vi "SerialFrameProtocol_example.vi"() -> ()   [LabVIEW 2015]
uses:
  <vilib>/Instr/_visa.llb/VISA Flush IO Buffer Mask.ctl
  <vilib>/Instr/_visa.llb/VISA Set IO Buffer Mask.ctl
  <vilib>/Instr/_visa.llb/VISA Configure Serial Port (Instr).vi
panel:
  out "length 2":i32
  out "length":i32
  in  "VISA resource name":refnum<visa-resource-name>="COM8"
  out "buffer, NORMAL == read buffer unstuffing, NORMAL":bool
  out "size(s)":i32
  out "size(s)":i32
  out "Receiv Array":u8[](array[numeric])
  out "Send Array":u8[](array[numeric])
  out "Data2 (U16)":u16[](array[numeric])
  out "size(Data2)":i32
  out "size(Data1)":i32
  out "Data1 (I32)":i32[](array[numeric])
  out "B0":cluster{"iVal":i32, "fVal":sgl}
  out "buffer, HEX":string
  out "buffer, NORMAL":string
  out "buffer stuffing, HEX":string
  in  "Clear log":bool
  in  "CA":bool
  out "log":string
  in  "CL":bool
  in  "CZ":bool
  out "VISA Read counter":i32
  out "error IO":errorcluster
  out "VISA Read no error counter":i32
  in  "CN":bool
  in  "CY":bool
  in  "CB":bool
  out "CX Send array == AX read array":bool
  out "read buffer unstuffing, HEX":string
  out "read buffer unstuffing, NORMAL":string
  out "buffer stuffing, NORMAL":string
  out "read buffer RAW, HEX":string
  in  "stop":bool
  out "Counter":i32
  out "read buffer RAW, NORMAL":string="\n"
  in  "CX Send rand array":bool
  # "Serial Frame Protocol Test"
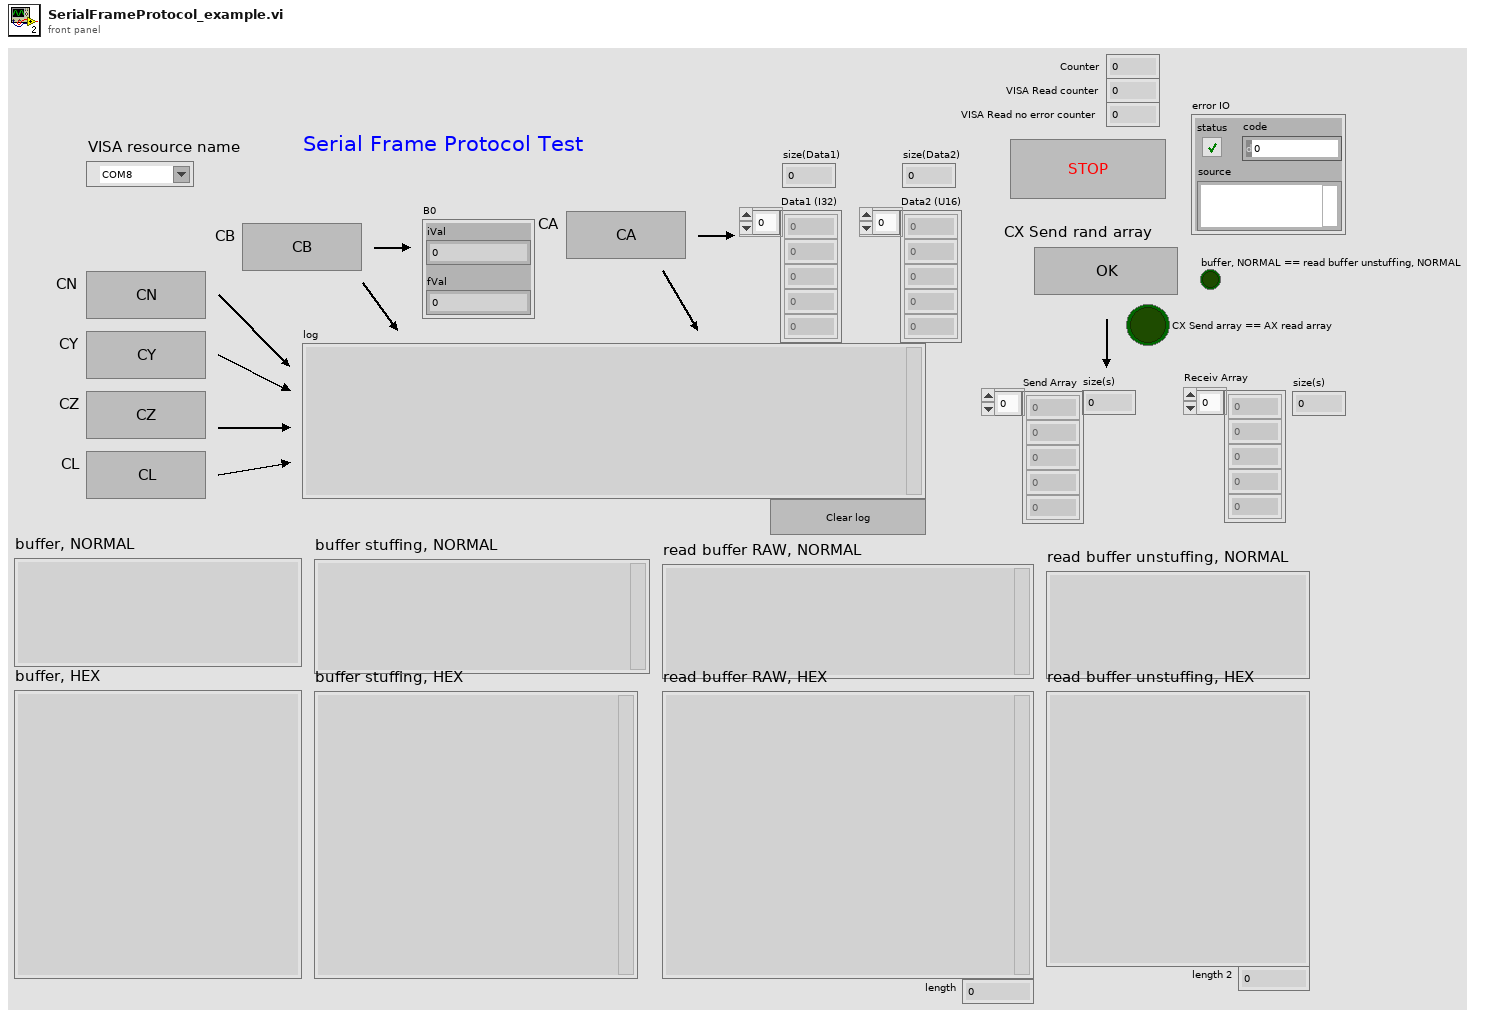
[diagram p1: front panel]
types:
  T1 = typedef "VISA Set IO Buffer Mask.ctl" = u16
  T2 = typedef "VISA Flush IO Buffer Mask.ctl" = u16
  T3 = enum16{"big-endian, network order", "native, host order", "little-endian"}
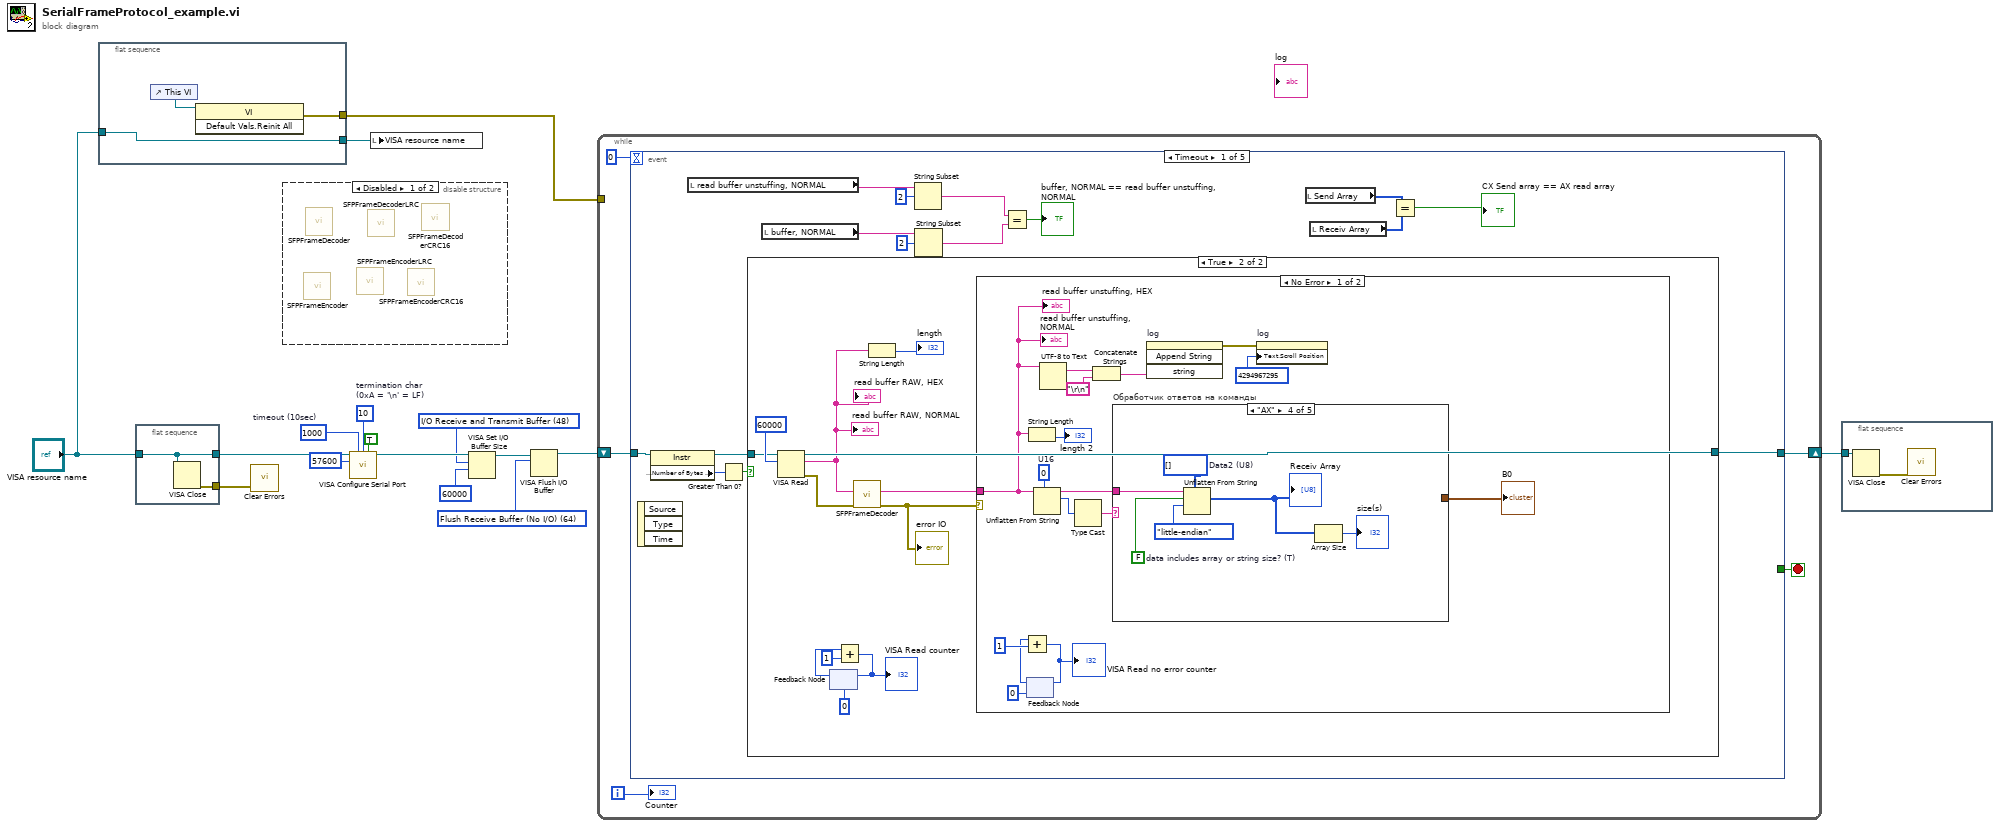
[diagram p0: block diagram]
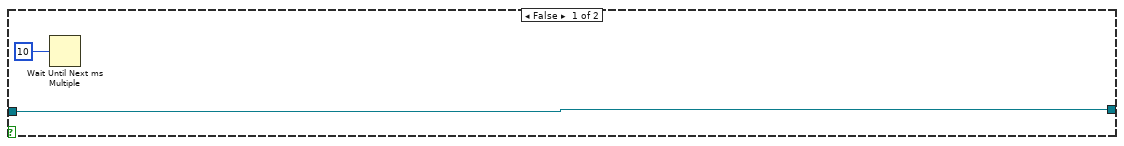
[diagram p2: hidden frame]
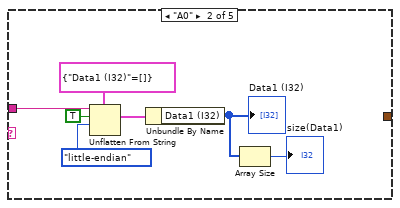
[diagram p4: hidden frame]
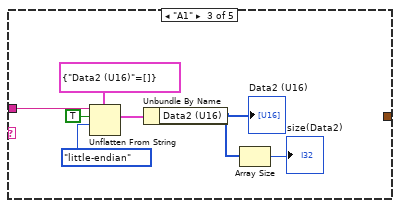
[diagram p5: hidden frame]
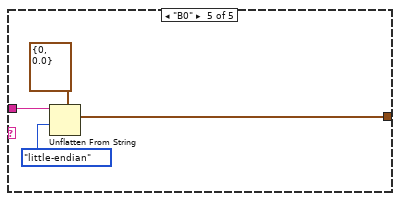
[diagram p6: hidden frame]
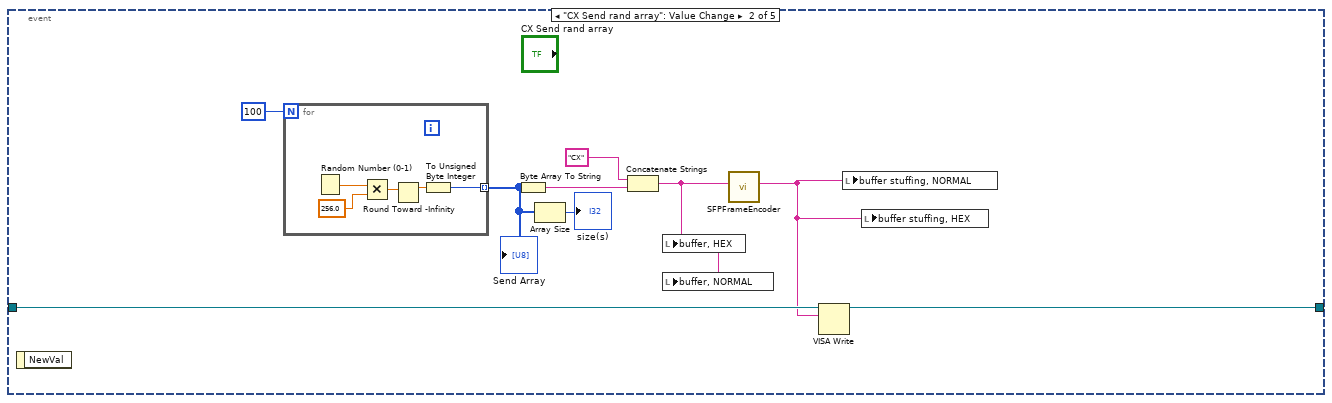
[diagram p8: hidden frame]
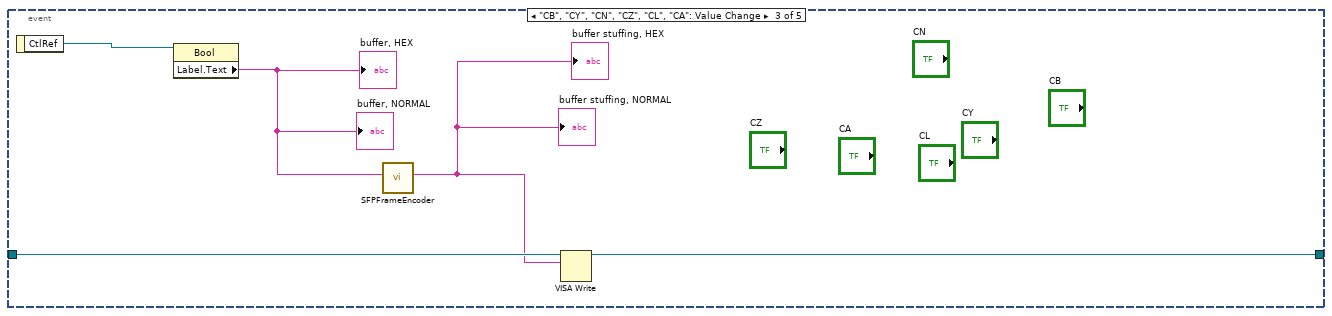
[diagram p9: hidden frame]
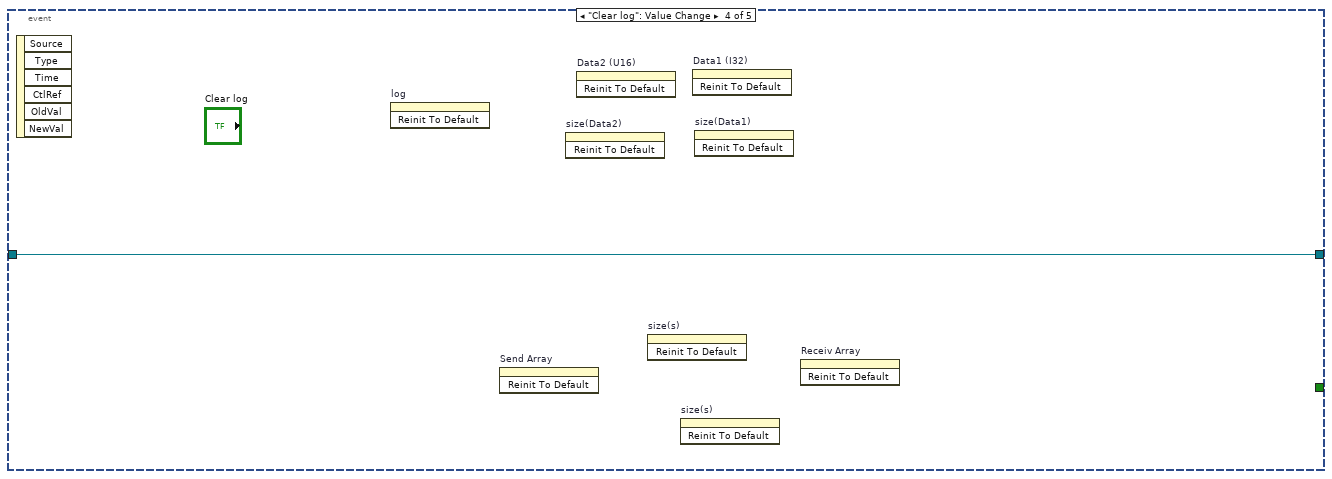
[diagram p10: hidden frame]
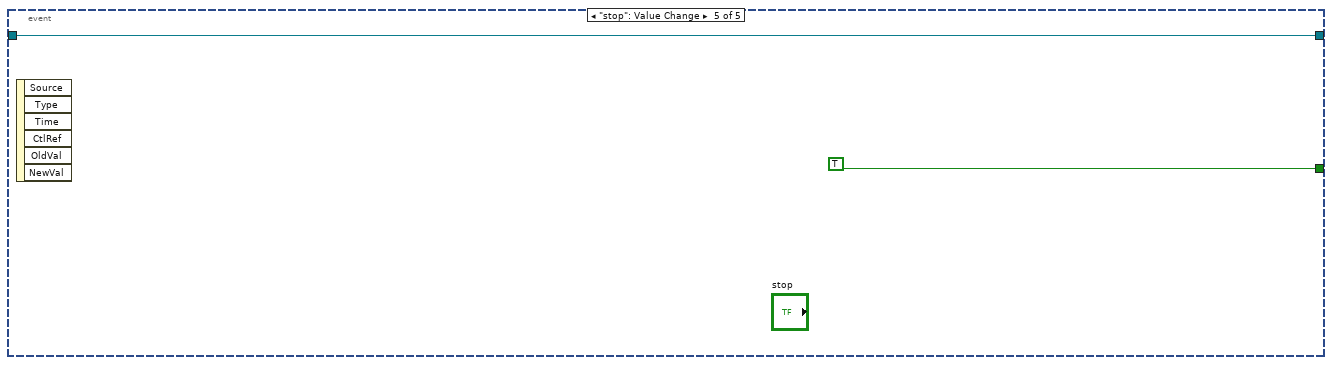
[diagram p11: hidden frame]
diagram:
  w5 = T1 48 items=["I/O Receive Buffer"=16, "I/O Transmit Buffer"=32, "I/O Receive and Transmit Buffer"=48] ("Mask")
  w7 = T2 64 items=["Flush Receive Buffer"=16, "Write Transmit Buffer to Device"=32, "Flush Receive Buffer (No I/O)"=64, "Flush Transmit Buffer"=128] ("Mask")
  w12 = u8 10  # termination char (0xA = '\n' = LF)
  w14 = u32 1000  # timeout (10sec)
  n1 = flat-sequence {
    tunnel: [w18] -> w8
    tunnel: "VISA resource name" -> [w17]
    tunnel: [w17] -> w1
    frame #0 {
      n2 = control-ref of="This VI"() -> (w19:refnum<vi>)
      n3 = invoke class="VI" method="Default Vals.Reinit All"(reference=w19) -> (error out=w18:errorcluster)  [unwired: 2 in, 2 out]
    }
  }
  n4 = flat-sequence {
    tunnel: "VISA resource name" -> [w21]
    tunnel: [w21] -> w10
    tunnel: [w20] -> w16
    frame #0 {
      n5 = VISA Close(VISA resource name=w21) -> (error out=w20:errorcluster)  [unwired: 1 in]
    }
  }
  n6 = call <vilib>:"Clear Errors.vi"("error in (no error)"=w16) -> ()  [unwired: 5 in, 2 out]
  n7 = disable-structure shown="Disabled" {
    frame Disabled {
      n8 = call-poly "SFPFrameEncoder.vi"() -> ()  [unwired: 4 in, 2 out]
      n9 = call-poly "SFPFrameDecoder.vi"() -> ()  [unwired: 6 in, 2 out]
      n10 = call "SFPFrameEncoderLRC.vi"() -> ()  [unwired: 4 in, 2 out]
      n11 = call "SFPFrameDecoderLRC.vi"() -> ()  [unwired: 6 in, 2 out]
      n12 = call "SFPFrameEncoderCRC16.vi"() -> ()  [unwired: 4 in, 2 out]
      n13 = call "SFPFrameDecoderCRC16.vi"() -> ()  [unwired: 6 in, 2 out]
    }
    frame Enabled {
    }
  }
  n14 = call-poly "VISA Configure Serial Port"("VISA resource name"=w10, "timeout (10sec)"=w14, "termination char\n(0xA = '\\n' = LF)"=w12, "Enable Termination\nChar (T)"=TRUE ("Enable Termination\nChar (T)"), "baud rate (9600)"=u32 57600) -> ("VISA resource name out"=w9:refnum<visa-resource-name>)  [unwired: 9 in, 1 out]
  n15 = local write "VISA resource name"(w1) -> ()
  n16 = VISA Set I/O Buffer Size(VISA resource name=w9, mask (16)=w5, size (4096)=u32 60000) -> (VISA resource name out=w6:refnum<visa-resource-name>)  [unwired: 1 in, 1 out]
  n17 = VISA Flush I/O Buffer(VISA resource name=w6, mask (16)=w7) -> (VISA resource name out=w3:refnum<visa-resource-name>)  [unwired: 1 in, 1 out]
  n18 = while {
    shift-right: [w22] -> w15
    shift-left: w3 -> [w23]
    tunnel: w8 -> [_]
    i -> [w24]
    stop <- w25 stop-if-true
    n19 = event shown="[0] Timeout" {
      selector: _ -> [_ _ _ _ _]
      dyn-events: _ -> [_ _ _ _ _]
      timeout: 0 -> [_ _ _ _ _]
      tunnel: [_ _ _ _ TRUE] -> w25
      tunnel: w23 -> [w38 w103 w113 w115 w116]
      tunnel: [w37 w102 w112 w115 w116] -> w22
      event Timeout {
        n20 = event-data() -> ()  [unwired: 1 in, 3 out]
        n21 = property class="Instr"(reference=w38) -> (reference out=w39:refnum<visa-resource-name>, "Serial Settings:Number of Bytes at Serial Port"=w40:u32)  [unwired: 1 in, 1 out]
        n22 = local read "read buffer unstuffing, NORMAL"() -> (w35:string)
        n23 = Greater Than 0?(x=w40) -> (x > 0?=w41:bool)
        n24 = case shown="True" w41 {
          tunnel: [w43 w50] -> w37
          tunnel: w39 -> [w43 w49]
          frame False {
            n25 = Wait Until Next ms Multiple(millisecond multiple=u32 10) -> ()  [unwired: 1 out]
          }
          frame True {
            n26 = VISA Read(VISA resource name=w49, byte count=u32 60000) -> (VISA resource name out=w50:refnum<visa-resource-name>, read buffer=w45:string, error out=w48:errorcluster)  [unwired: 1 in, 1 out]
            "read buffer RAW, NORMAL" <- w45
            "read buffer RAW, HEX" <- w45
            n27 = feedback #1(0) -> (w52:i32)
            n28 = Add(x=w52, y=1) -> (x+y=w53:i32)
            "VISA Read counter" <- w53
            n29 = feedback-in #1(w53) -> ()
            n30 = call-poly "SFPFrameDecoder.vi"("error in (no error)"=w48, "Encoded frame"=w45) -> ("error out"=w46:errorcluster, "Decoded data"=w47:string)  [unwired: 4 in]
            "error IO" <- w46
            n31 = String Length(string=w45) -> (length=→"length":i32)
            n32 = case shown="No Error" w46 {
              tunnel: w47 -> [w57 _]
              frame No Error {
                w62 = u16 0  # U16
                n33 = feedback #2(0) -> (w70:i32)
                n34 = Add(x=w70, y=1) -> (x+y=w69:i32)
                "VISA Read no error counter" <- w69
                n35 = feedback-in #2(w69) -> ()
                n36 = String Length(string=w57) -> (length=→"length 2":i32)
                n37 = Unflatten From String(type=w62, binary string=w57) -> (rest of the binary string=w59:string, value=w60:u16)  [unwired: 3 in, 1 out]
                n38 = UTF-8 to Text(11:w57) -> (3:w63:string)  [unwired: 2 in, 1 out]
                n39 = Type Cast(x=w60) -> (*(type *) &x=w61:string)  [unwired: 1 in]
                n40 = Concatenate Strings(w63, "\r\n") -> (w65:string)
                n41 = case "Обработчик ответов на команды" shown="\"AX\"" w61 {
                  tunnel: w59 -> [_ w76 w83 w90 w93]
                  tunnel: [_ _ _ _ w92] -> w58
                  frame Default {
                    # "Пустой обрабтчик"
                  }
                  frame "A0" {
                    n42 = Unflatten From String(type=cluster{"Data1 (I32)":i32[]} {"Data1 (I32)"=[]}, binary string=w76, data includes array or string size? (T)=TRUE, byte order (0:big-endian, network order)=T3."little-endian") -> (value=w74:cluster{"Data1 (I32)":i32[]})  [unwired: 1 in, 2 out]
                    n43 = Unbundle By Name(w74) -> ("Data1 (I32)"=w73:i32[])
                    "Data1 (I32)" <- w73
                    n44 = Array Size(array=w73) -> (size(s)=→"size(Data1)":i32)
                  }
                  frame "A1" {
                    n45 = Unflatten From String(type=cluster{"Data2 (U16)":u16[]} {"Data2 (U16)"=[]}, binary string=w83, data includes array or string size? (T)=TRUE, byte order (0:big-endian, network order)=T3."little-endian") -> (value=w81:cluster{"Data2 (U16)":u16[]})  [unwired: 1 in, 2 out]
                    n46 = Unbundle By Name(w81) -> ("Data2 (U16)"=w80:u16[])
                    "Data2 (U16)" <- w80
                    n47 = Array Size(array=w80) -> (size(s)=→"size(Data2)":i32)
                  }
                  frame "AX" {
                    w87 = u8[] []  # Data2 (U8)
                    w89 = FALSE  # data includes array or string size? (T)
                    n48 = Unflatten From String(type=w87, binary string=w90, data includes array or string size? (T)=w89, byte order (0:big-endian, network order)=T3."little-endian") -> (value=w86:u8[])  [unwired: 1 in, 2 out]
                    "Receiv Array" <- w86
                    n49 = Array Size(array=w86) -> (size(s)=→"size(s)":i32)
                  }
                  frame "B0" {
                    n50 = Unflatten From String(type=cluster{"iVal":i32, "fVal":sgl} {"iVal"=0, "fVal"=0.0}, binary string=w93, byte order (0:big-endian, network order)=T3."little-endian") -> (value=w92:cluster{"iVal":i32, "fVal":sgl})  [unwired: 2 in, 2 out]
                  }
                }
                "B0" <- w58
                n51 = invoke on="log" class="Str" method="Append String"("string"=w65) -> (error out=w66:errorcluster)  [unwired: 3 in, 3 out]
                n52 = property on="log" class="Str"(error in=w66, "Text.Scroll Position"=u32 4294967295) -> ()  [unwired: 1 in, 2 out]
                "read buffer unstuffing, HEX" <- w57
                "read buffer unstuffing, NORMAL" <- w57
              }
              frame Error {
              }
            }
          }
        }
        n53 = local read "buffer, NORMAL"() -> (w33:string)
        n54 = String Subset(string=w35, offset (0)=2) -> (substring=w32:string)  [unwired: 1 in]
        n55 = String Subset(string=w33, offset (0)=2) -> (substring=w31:string)  [unwired: 1 in]
        n56 = Equal?(x=w32, y=w31) -> (x = y?=→"buffer, NORMAL == read buffer unstuffing, NORMAL":bool)
        n57 = local read "Send Array"() -> (w30:u8[])
        n58 = local read "Receiv Array"() -> (w29:u8[])
        n59 = Equal?(x=w30, y=w29) -> (x = y?=→"CX Send array == AX read array":bool)
      }
      event "CX Send rand array": Value Change {
        n60 = event-data() -> ()  [unwired: 1 in, 1 out]
        n61 = for {
          N: 100 -> [_]
          tunnel: [w105] -> w97 mode=indexing
          n62 = Random Number (0-1)() -> (number: 0 to 1=w109:dbl)
          n63 = Multiply(x=w109, y=256.0) -> (x*y=w107:dbl)
          n64 = Round Toward -Infinity(1:w107) -> (0:w106:dbl)
          n65 = To Unsigned Byte Integer(number=w106) -> (unsigned 8bit integer=w105:u8)
        }
        "Send Array" <- w97
        n66 = Byte Array To String(unsigned byte array=w97) -> (string=w99:string)
        n67 = Array Size(array=w97) -> (size(s)=→"size(s)":i32)
        n68 = Concatenate Strings("CX" ("string"), w99) -> (w98:string)
        n69 = local write "buffer, HEX"(w98) -> ()
        n70 = local write "buffer, NORMAL"(w98) -> ()
        n71 = call-poly "SFPFrameEncoder.vi"("Data"=w98) -> ("Encoded frame"=w100:string)  [unwired: 5 in, 1 out]
        n72 = VISA Write(VISA resource name=w103, write buffer=w100) -> (VISA resource name out=w102:refnum<visa-resource-name>)  [unwired: 1 in, 2 out]
        n73 = local write "buffer stuffing, NORMAL"(w100) -> ()
        n74 = local write "buffer stuffing, HEX"(w100) -> ()
      }
      event "CB", "CY", "CN", "CZ", "CL", "CA": Value Change {
        n75 = event-data() -> ("CtlRef"=w114:refnum<vi>)  [unwired: 1 in]
        n76 = property class="Bool"(reference=w114) -> ("Label.Text"=w110:string)  [unwired: 1 in, 2 out]
        "buffer, NORMAL" <- w110
        "buffer, HEX" <- w110
        n77 = call-poly "SFPFrameEncoder.vi"("Data"=w110) -> ("Encoded frame"=w111:string)  [unwired: 5 in, 1 out]
        "buffer stuffing, HEX" <- w111
        "buffer stuffing, NORMAL" <- w111
        n78 = VISA Write(VISA resource name=w113, write buffer=w111) -> (VISA resource name out=w112:refnum<visa-resource-name>)  [unwired: 1 in, 2 out]
      }
      event "Clear log": Value Change {
        n79 = event-data() -> ()  [unwired: 1 in, 6 out]
        n80 = invoke on="log" class="Str" method="Reinit To Default"() -> ()  [unwired: 3 in, 3 out]
        n81 = invoke on="Send Array" class="Arr (strict)" method="Reinit To Default"() -> ()  [unwired: 3 in, 3 out]
        n82 = invoke on="size(Data2)" class="DigNum (strict)" method="Reinit To Default"() -> ()  [unwired: 3 in, 3 out]
        n83 = invoke on="Data2 (U16)" class="Arr (strict)" method="Reinit To Default"() -> ()  [unwired: 3 in, 3 out]
        n84 = invoke on="size(s)" class="DigNum (strict)" method="Reinit To Default"() -> ()  [unwired: 3 in, 3 out]
        n85 = invoke on="size(s)" class="DigNum (strict)" method="Reinit To Default"() -> ()  [unwired: 3 in, 3 out]
        n86 = invoke on="Data1 (I32)" class="Arr (strict)" method="Reinit To Default"() -> ()  [unwired: 3 in, 3 out]
        n87 = invoke on="size(Data1)" class="DigNum (strict)" method="Reinit To Default"() -> ()  [unwired: 3 in, 3 out]
        n88 = invoke on="Receiv Array" class="Arr (strict)" method="Reinit To Default"() -> ()  [unwired: 3 in, 3 out]
      }
      event "stop": Value Change {
        n89 = event-data() -> ()  [unwired: 1 in, 6 out]
      }
    }
    "Counter" <- w24
  }
  n90 = flat-sequence {
    tunnel: w15 -> [w119]
    frame #0 {
      n91 = VISA Close(VISA resource name=w119) -> (error out=w118:errorcluster)  [unwired: 1 in]
      n92 = call <vilib>:"Clear Errors.vi"("error in (no error)"=w118) -> ()  [unwired: 5 in, 2 out]
    }
  }
